vi "test_pid_output.vi"() -> ()   [LabVIEW 2018]
uses:
  FPGA/PID/PID control enabled type.ctl
  <vilib>/rvi/Emulation/niFpgaSctlEmulationGetInTimedLoop.vi
  <vilib>/rvi/Memory/Memory_Emulation/nirvimemoryFastEmulation.vi
  <vilib>/rvi/Memory/Memory_Emulation/nirvimemoryEmulation.vi
  <vilib>/rvi/Emulation/niFpgaEmulationIsFPGAContextNoSignature.vi
  <vilib>/rvi/DataTransferAndStorage/Container/Common/niFpgaContainerGetUniqueNameForEmu.vi
  <vilib>/rvi/Emulation/niFpgaProcessEmulError.vi
  <vilib>/rvi/errors/nirviReportUnexpectedCaseInternalError (U32).vi
  <vilib>/rvi/DataTransferAndStorage/Container/XNode/niFpgaContainer.xnode
panel:
  out "Waveform Graph 3":i16[][](graph)
  out "Waveform Graph 2":dbl[][](graph)
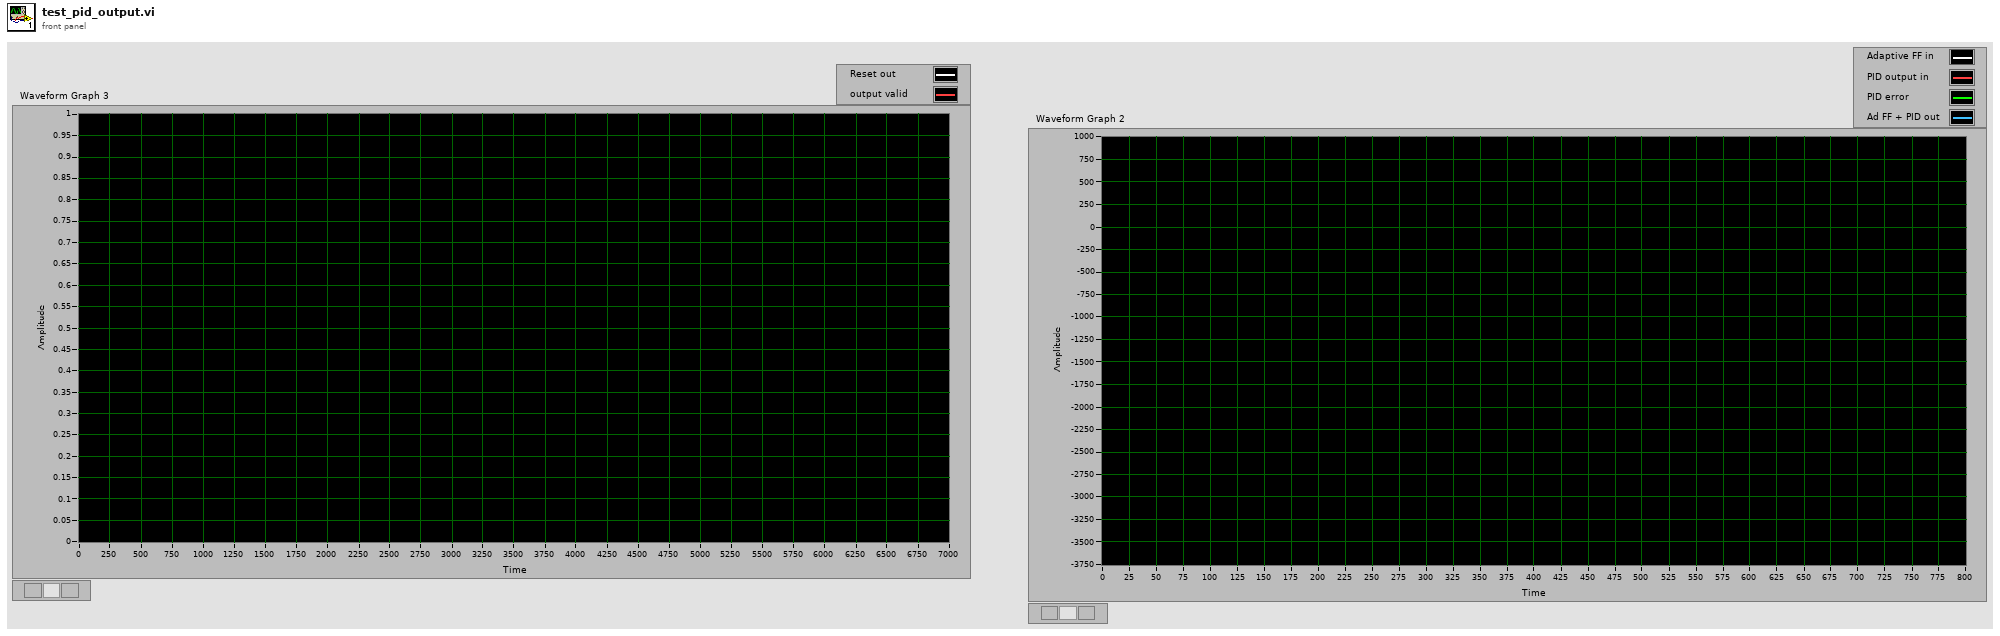
[diagram p1: front panel]
types:
  T1 = typedef "PID control enabled type.ctl" = enum16{"PID on", "Ref", "Zero"}
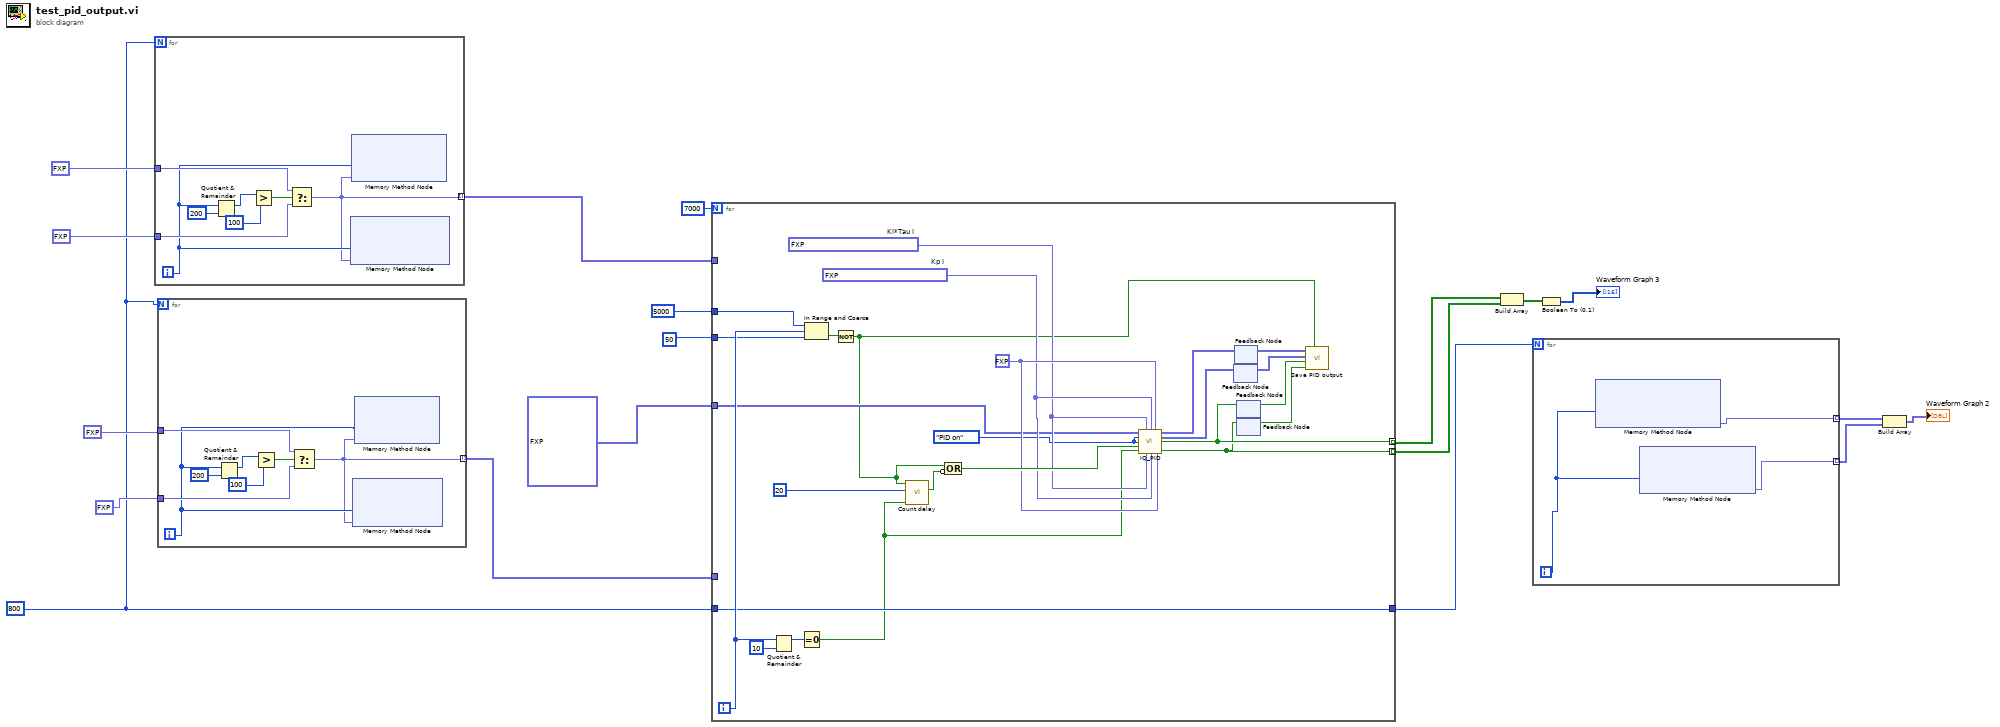
[diagram p0: block diagram]
diagram:
  w11 = u32 800 ("Data")
  n1 = for {
    N: w11 -> [_]
    tunnel: fxp<+/-,32,14> 100.0 ("Data") -> [w23]
    tunnel: fxp<+/-,32,14> 500.0 ("Data") -> [w22]
    tunnel: [w20] -> w9 mode=indexing
    i -> [w21]
    n2 = Quotient & Remainder(x=w21, y=200) -> (x-y*floor(x/y)=w26:i32)  [unwired: 1 out]
    n3 = Greater?(x=w26, y=100) -> (0:w24:bool)
    n4 = Select(t=w23, s=w24, f=w22) -> (s? t:f=w20:fxp<+/-,32,14>)
    n5 = xnode ("Memory Method Node")("Address"=w21, "Data"=w20) -> ()  [unwired: 1 in, 1 out]
    n6 = xnode ("Memory Method Node")("Address"=w21, "Data"=w20) -> ()  [unwired: 1 in, 1 out]
  }
  n7 = for {
    N: w11 -> [_]
    tunnel: fxp<+/-,32,14> 800.0 ("Data") -> [w32]
    tunnel: fxp<+/-,32,14> 400.0 ("Data") -> [w31]
    tunnel: [w29] -> w10 mode=indexing
    i -> [w30]
    n8 = Quotient & Remainder(x=w30, y=200) -> (x-y*floor(x/y)=w34:i32)  [unwired: 1 out]
    n9 = Greater?(x=w34, y=100) -> (0:w28:bool)
    n10 = Select(t=w32, s=w28, f=w31) -> (s? t:f=w29:fxp<+/-,32,14>)
    n11 = xnode ("Memory Method Node")("Address"=w30, "Data"=w29) -> ()  [unwired: 1 in, 1 out]
    n12 = xnode ("Memory Method Node")("Address"=w30, "Data"=w29) -> ()  [unwired: 1 in, 1 out]
  }
  n13 = for {
    N: 7000 -> [_]
    tunnel: [w36] -> w3 mode=indexing
    tunnel: [w37] -> w4 mode=indexing
    tunnel: 50 ("y") -> [w50]
    tunnel: 5000 ("y") -> [w49]
    tunnel: fxp<+/-,32,14>[] [1000.0, 1000.0, 2000.0, 2000.0] ("Data in") -> [w47]
    tunnel: w11 -> [w40]
    tunnel: w10 -> [_]
    tunnel: w9 -> [_]
    tunnel: [w40] -> w6
    i -> [w51]
    w52 = PID_control_enabled_type."PID on" ("Enable Q")
    w53 = fxp<+/-,32,6> 0.01000000536441803  # Ki*Tau I
    w54 = fxp<+/-,32,6> 0.1000000536441803  # Kp I
    w55 = fxp<+/-,32,6> 0.0 ("Kd/Tau I")
    n14 = Quotient & Remainder(x=w51, y=10) -> (x-y*floor(x/y)=w57:i32)  [unwired: 1 out]
    n15 = Equal To 0?(x=w57) -> (x = 0?=w39:bool)
    n16 = In Range and Coerce(upper limit=w49, x=w51, lower limit=w50) -> (In Range?=w48:bool)  [unwired: 1 out]
    n17 = Not(x=w48) -> (.not. x?=w38:bool)
    n18 = call "Count delay.vi"("input valid"=w39, "Count to skip"=u32 20, "Reset"=w38) -> ("count done?"=w60:bool)  [unwired: 7 in, 1 out]
    n19 = Compound Arithmetic op=OR(w38, invert w60) -> (w59:bool)
    n20 = call "IQ_PID.vi"("Data in"=w47, "Ki*Tau I"=w53, "Kp I"=w54, "Kd/Tau I"=w55, "Enable I"=w52, "Enable Q"=w52, "Reset"=w59, "input valid"=w39, "Ki*Tau Q"=w53, "Kp Q"=w54, "Kd/Tau Q"=w55) -> ("data out"=w46:fxp<+/-,32,14>[], "e(n) out"=w44:fxp<+/-,32,14>[], "Reset out"=w37:bool, "output valid"=w36:bool)  [unwired: 1 in]
    n21 = feedback #1() -> (w43:fxp<+/-,32,14>[])  [unwired: 1 in]
    n22 = feedback-in #1(w44) -> ()
    n23 = feedback #2() -> (w45:fxp<+/-,32,14>[])  [unwired: 1 in]
    n24 = feedback-in #2(w46) -> ()
    n25 = feedback #3() -> (w42:bool)  [unwired: 1 in]
    n26 = feedback-in #3(w37) -> ()
    n27 = feedback #4() -> (w41:bool)  [unwired: 1 in]
    n28 = feedback-in #4(w36) -> ()
    n29 = call "Save PID output.vi"("Reset"=w38, "input valid"=w41, "Write zero"=w42, "e(n) in"=w43, "Data in"=w45) -> ()  [unwired: 7 in]
  }
  n30 = Build Array(w4, w3) -> (w2:bool[][])
  n31 = for {
    N: w6 -> [_]
    tunnel: [w61] -> w8 mode=indexing
    tunnel: [w62] -> w5 mode=indexing
    i -> [w63]
    n32 = xnode ("Memory Method Node")("Address"=w63) -> ("Data"=w62:fxp<+/-,32,14>)  [unwired: 1 in, 1 out]
    n33 = xnode ("Memory Method Node")("Address"=w63) -> ("Data"=w61:fxp<+/-,32,14>)  [unwired: 1 in, 1 out]
  }
  n34 = Boolean To (0,1)(Boolean=w2) -> (0, 1=→"Waveform Graph 3":i16[][])
  n35 = Build Array(w5, w8) -> (→"Waveform Graph 2":fxp<+/-,32,14>[][])
